vi "shifter.vi"(2 "Solenoids":bool[](array[boolean])=[FALSE, FALSE, FALSE, FALSE, FALSE, FALSE, FALSE, FALSE], 3 "CurrentStatusArray":bool[][](array[boolean]), 4 "Checkmarks LED array":bool[][](array[boolean])) -> (0 "outputCurrentStatusArray":bool[][](array[boolean]), 1 "outputCheckmarksArray":bool[][](array[boolean]))   [LabVIEW 2011]
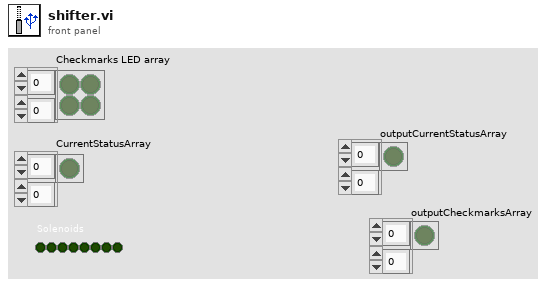
[diagram p1: front panel]
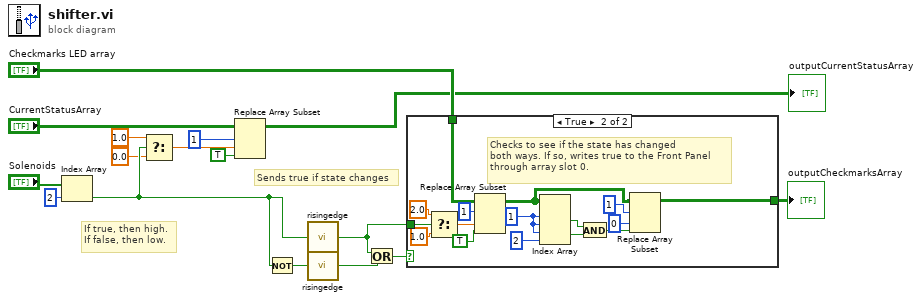
[diagram p0: block diagram]
diagram:
  # "Sends true if state changes"
  # "If true, then high.\nIf false, then low."
  n1 = Index Array(array="Solenoids", index=2) -> (element=w5:bool)
  n2 = Select(t=1.0, s=w5, f=0.0) -> (s? t:f=w1:dbl)
  n3 = Replace Array Subset(array="CurrentStatusArray", new element=TRUE ("new element/subarray"), index (row)=1, index (col)=w1) -> (→"outputCurrentStatusArray":bool[][])
  n4 = Not(x=w5) -> (.not. x?=w7:bool)
  n5 = call "risingedge.vi"("Input"=w5) -> ("Output"=w8:bool)
  n6 = call "risingedge.vi"("Input"=w7) -> ("Output"=w6:bool)
  n7 = Or(x=w8, y=w6) -> (x .or. y?=w11:bool)
  n8 = case shown="True" w11 {
    tunnel: "Checkmarks LED array" -> [w17 w30]
    tunnel: [w17 w18] -> w9
    tunnel: w8 -> [_ w33]
    frame False {
    }
    frame True {
      w25 = 1 ("index (row)")
      # "Checks to see if the state has changed\nboth ways. If so, writes true to the Front Panel\nthrough array slot 0."
      n9 = Select(t=2.0, s=w33, f=1.0) -> (s? t:f=w29:dbl)
      n10 = Replace Array Subset(array=w30, new element=TRUE ("new element/subarray"), index (row)=1 ("disabled index (row)"), index (col)=w29) -> (w21:bool[][])
      n11 = Index Array(array=w21, index (row) #1=w25, index (col) #1=w25, index (row) #2=w25, index (col) #2=2 ("disabled index (col)")) -> (element #1=w24:bool, element #2=w23:bool)
      n12 = And(x=w24, y=w23) -> (x .and. y?=w22:bool)
      n13 = Replace Array Subset(array=w21, new element=w22, index (row)=1, index (col)=0 ("disabled index (col)")) -> (w18:bool[][])
    }
  }
  "outputCheckmarksArray" <- w9
